vi "Actor Core.vi"(8 "error in":errorcluster, 11 "Batch proc":refnum<class "Batch Processor.lvclass">) -> (0 "error out":errorcluster, 3 "Actor out":refnum<class "Actor.lvclass">)   [LabVIEW 2016, in "Batch Processor.lvclass"]
doc: "LabActor main control pannel"
uses:
  Batch Processor.lvclass
  C:/Github/LabActor/Controllers/Application Controller/Application Controller.lvclass
  C:/Github/LabActor/Template Module/Template Module.lvclass
  C:/Program Files/National Instruments/LabVIEW 2016/vi.lib/ActorFramework/Actor/Actor.lvclass
  <vilib>/ActorFramework/Actor/Actor.lvclass
  NHMFL_Core/Libraries/Queued Listbox/Queued Listbox.xctl
  Application Controller/Application Controller.lvclass/Application Controller.ctl
  Template Module/Template Module.lvclass/Template Module.ctl
  <vilib>/ActorFramework/Actor/Actor.lvclass/Actor.ctl
  <vilib>/ActorFramework/Message Enqueuer/Message Enqueuer.lvclass/Message Enqueuer.ctl
  Batch Processor Messages/Start Batch Process Msg/Start Batch Process Msg.lvclass/Start Batch Process Msg.ctl
  <vilib>/Utility/sysdir.llb/System Directory Type.ctl
  Template Module Messages/Save Configuration Msg/Save Configuration Msg.lvclass/Save Configuration Msg.ctl
  Batch Processor Messages/List Folder Files Msg/List Folder Files Msg.lvclass/List Folder Files Msg.ctl
  Plots/Plot types.ctl
  Application Controller Messages/Open Waveform File Plot Msg/Open Waveform File Plot Msg.lvclass/Open Waveform File Plot Msg.ctl
  Monitor-Pulse Messages/Stop Measurements Command Msg/Stop Measurements Command Msg.lvclass/Stop Measurements Command Msg.ctl
  Application Controller/Write Monitor Running.vi
  Application Controller/Write Monitor ref.vi
  Application Controller/Write Start button.vi
  Application Controller/Write Stop button.vi
  Template Module/Read stop event.vi
  Application Controller/Read Monitor start event.vi
  Application Controller/Read Monitor stop event.vi
  Template Module/Read Open item event.vi
  Application Controller/Write Postproc ref.vi
  <vilib>/ActorFramework/Message Enqueuer/Init from Existing Queue.vi
  <vilib>/ActorFramework/Message Enqueuer/Enqueue.vi
  <vilib>/ActorFramework/Stop Msg/Stop Msg.lvclass
  C:/Program Files/National Instruments/LabVIEW 2016/vi.lib/ActorFramework/Message/Message.lvclass
  Batch Processor Messages/Start Batch Process Msg/Start Batch Process Msg.lvclass
  Template Module Messages/Save Configuration Msg/Save Configuration Msg.lvclass
  Batch Processor Messages/List Folder Files Msg/List Folder Files Msg.lvclass
  Application Controller Messages/Open Waveform File Plot Msg/Open Waveform File Plot Msg.lvclass
  Monitor-Pulse Messages/Stop Measurements Command Msg/Stop Measurements Command Msg.lvclass
  <vilib>/ActorFramework/Message Priority Queue/Priority Enqueue.vi
  Application Controller/Application Controller.lvclass
  <vilib>/ActorFramework/Message Enqueuer/Message Enqueuer.lvclass
  Template Module Messages/Restore Configuration Msg/Restore Configuration Msg.lvclass
panel:
  out "Elapsed time":dbl format="%#_gs"
  in  "Configuration":T1
  in  "All files in folder":bool
  in  "About Button":bool
  in  "Clear log":bool
  out "Error log":string
  out "Monitor file":path caption="Monitor\nFile"
  in  "Exit":bool
  in  "Write cfg":bool
  in  "Read cfg":bool
  in  "View XY Plot":bool
  out "Monitor Running":bool
  in  "Stop monitor":bool
  in  "Start monitor":bool
  in  "Monitor":string[](xcontrol) caption="Processors"
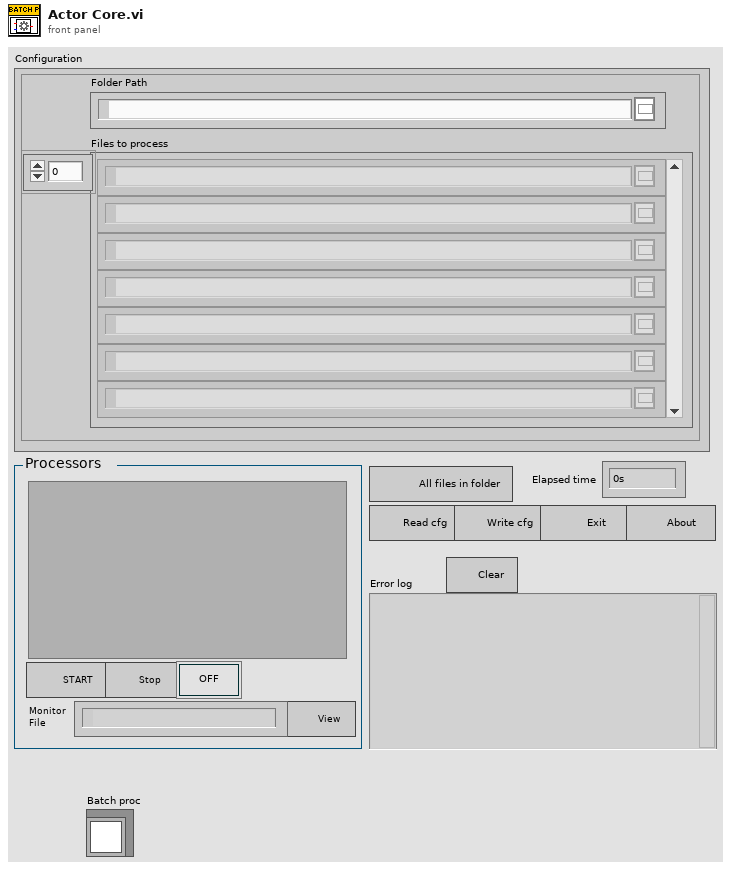
[diagram p1: front panel]
types:
  T1 = cluster{"Folder Path":path, "Files to process":path[]}
  T2 = typedef "Plot types.ctl" = enum16{"Waveform Plot", "XY Plot", "Full XY"}
  T3 = typedef "System Directory Type.ctl" = i32
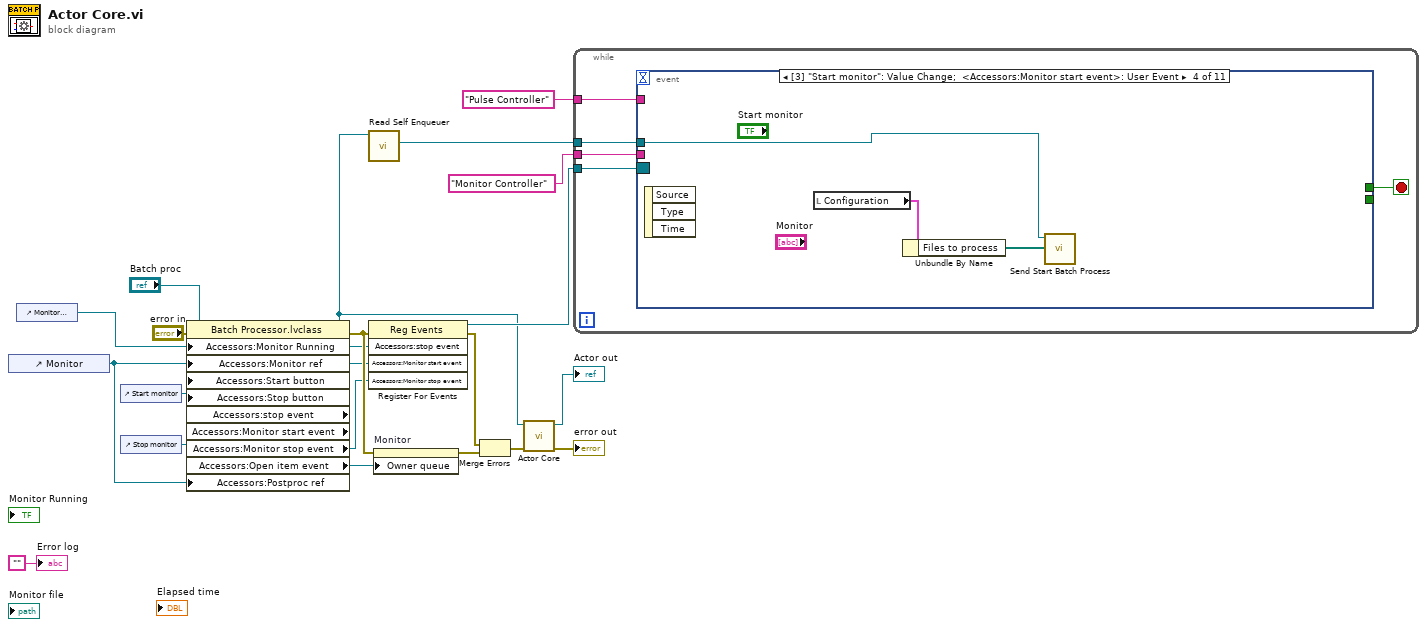
[diagram p0: block diagram]
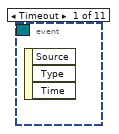
[diagram p2: hidden frame]
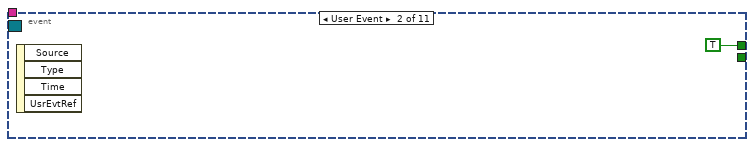
[diagram p3: hidden frame]
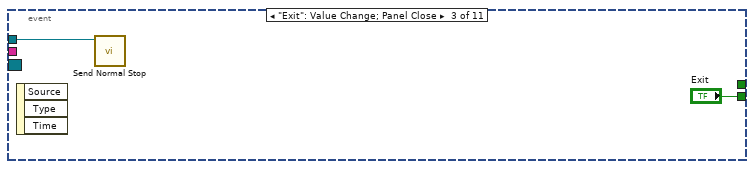
[diagram p4: hidden frame]
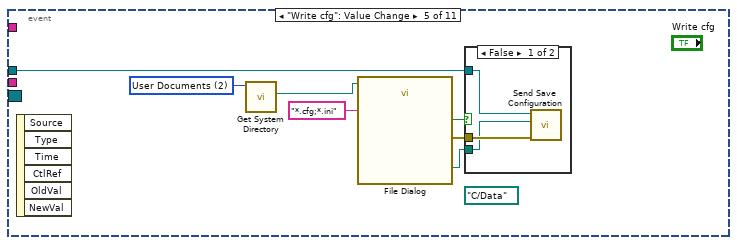
[diagram p5: hidden frame]
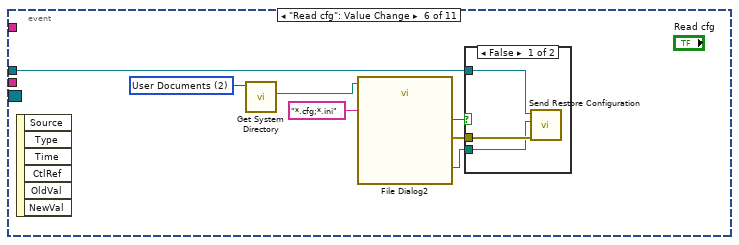
[diagram p7: hidden frame]
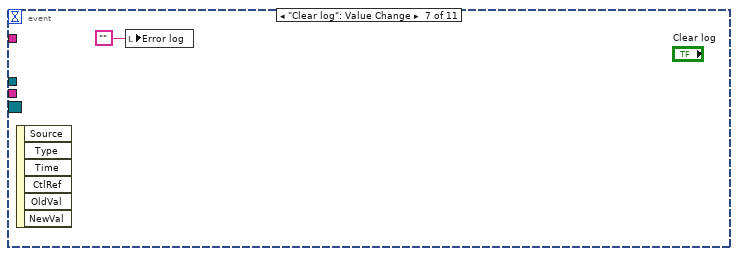
[diagram p9: hidden frame]
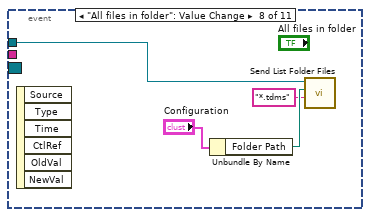
[diagram p10: hidden frame]
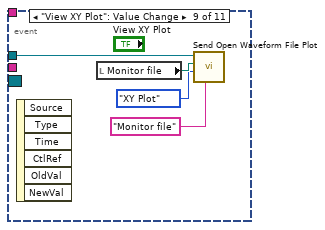
[diagram p11: hidden frame]
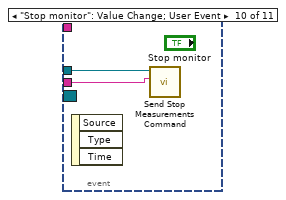
[diagram p12: hidden frame]
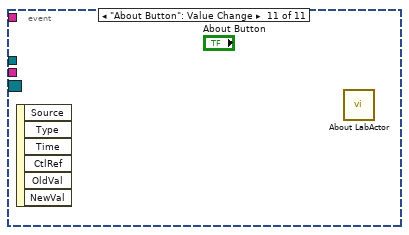
[diagram p13: hidden frame]
diagram:
  n1 = control-ref of="Monitor"() -> (w1:refnum<vi>)
  n2 = control-ref of="Monitor Running"() -> (w6:refnum<vi>)
  n3 = control-ref of="Start monitor"() -> (w4:refnum<vi>)
  n4 = control-ref of="Stop monitor"() -> (w5:refnum<vi>)
  n5 = property class="Batch Processor.lvclass"(reference="Batch proc", error in="error in", "Accessors:Monitor Running"=w6, "Accessors:Monitor ref"=w1, "Accessors:Start button"=w4, "Accessors:Stop button"=w5, "Accessors:Postproc ref"=w1) -> (reference out=w12:refnum<class "Batch Processor.lvclass">, error out=w16:errorcluster, "Accessors:stop event"=w7:refnum<user-event>, "Accessors:Monitor start event"=w3:refnum<user-event>, "Accessors:Monitor stop event"=w2:refnum<user-event>, "Accessors:Open item event"=w18:refnum<user-event>)
  n6 = call <vilib>:"Read Self Enqueuer.vi"("Actor"=w12) -> ("Self Enqueuer"=w11:refnum<class "Message Enqueuer.lvclass">)  [unwired: 10 in]
  n7 = register-events(error in=w16, w7, w3, w2) -> (reference out=w19:refnum<event-registration>, error out=w15:errorcluster)  [unwired: 1 in]
  n8 = property on="Monitor" class="Queued Listbox (strict)"(error in=w16, "Owner queue"=w18) -> (error out=w17:errorcluster)  [unwired: 1 in, 1 out]
  n9 = Merge Errors(w15, w17) -> (w13:errorcluster)
  n10 = call-parent "Actor Core.vi"("error in"=w13, "Measure Object in"=w12) -> ("error out"=→"error out":errorcluster, "Actor out"=→"Actor out":refnum<class "Actor.lvclass">)  [unwired: 8 in]
  n11 = while {
    tunnel: w19 -> [w27]
    tunnel: w11 -> [w25]
    tunnel: "Monitor Controller" ("Controller name") -> [w24]
    tunnel: "Pulse Controller" ("Item name") -> [w23]
    stop <- w26 stop-if-true
    n12 = event shown="[3] \"Start monitor\": Value Change;  <Accessors:Monitor start event>: User Event" {
      selector: w27 -> [_ _ _ _ _ _ _ _ _ _ _]
      dyn-events: _ -> [_ _ _ _ _ _ _ _ _ _ _]
      timeout: _ -> [_ _ _ _ _ _ _ _ _ _ _]
      tunnel: [_ TRUE _ _ _ _ _ _ _ _ _] -> w26
      tunnel: w25 -> [_ _ w29 w33 w37 w45 _ w58 w62 w64 _]
      tunnel: [_ _ "Exit" _ _ _ _ _ _ _ _] -> _
      tunnel: w24 -> [_ _ _ _ _ _ _ _ _ w63 _]
      tunnel: w23 -> [_ _ _ _ _ _ _ _ _ _ _]
      event Timeout {
        n13 = event-data() -> ()  [unwired: 1 in, 3 out]
      }
      event User Event {
        n14 = event-data() -> ()  [unwired: 1 in, 4 out]
      }
      event "Exit": Value Change; Panel Close {
        n15 = event-data() -> ()  [unwired: 1 in, 3 out]
        n16 = call <vilib>:"Send Normal Stop.vi"("Message Enqueuer"=w29) -> ()  [unwired: 10 in, 1 out]
      }
      event "Start monitor": Value Change; User Event {
        n17 = event-data() -> ()  [unwired: 1 in, 3 out]
        n18 = local read "Configuration"() -> (w32:T1)
        n19 = Unbundle By Name(w32) -> ("Files to process"=w31:path[])
        n20 = call "Send Start Batch Process.vi"("Files to process"=w31, "Message Enqueuer"=w33) -> ()  [unwired: 8 in, 2 out]
      }
      event "Write cfg": Value Change {
        w35 = T3 2 items=["User Home"=0, "User Desktop"=1, "User Documents"=2, "User Application Data"=3, "User Preferences"=4, "User Temporary"=5, "Public Documents"=6, "Public Application Data"=7, "Public Preferences"=8, "Public Cache"=13, "System Core Libraries"=9, "System Installed Libraries"=10, "Application Files"=11, "Boot Volume Root"=12] ("system directory type")
        (unwired) path "C:/Data" ("start path")
        n21 = event-data() -> ()  [unwired: 1 in, 6 out]
        n22 = call <vilib>:"Get System Directory.vi"("system directory type"=w35) -> ("system directory"=w34:path)  [unwired: 10 in]
        n23 = call "File Dialog"("start path"=w34, "pattern (all files)"="*.cfg;*.ini") -> ("selected path"=w39:path, "cancelled"=w40:bool, "error out"=w36:errorcluster)  [unwired: 10 in, 1 out]
        n24 = case shown="False" w40 {
          tunnel: w39 -> [w41 _]
          tunnel: w37 -> [w43 _]
          tunnel: w36 -> [w42 _]
          frame False {
            n25 = call "Send Save Configuration.vi"("error in (no error)"=w42, "File path"=w41, "Message Enqueuer"=w43) -> ()  [unwired: 7 in, 2 out]
          }
          frame True {
          }
        }
      }
      event "Read cfg": Value Change {
        w47 = T3 2 items=["User Home"=0, "User Desktop"=1, "User Documents"=2, "User Application Data"=3, "User Preferences"=4, "User Temporary"=5, "Public Documents"=6, "Public Application Data"=7, "Public Preferences"=8, "Public Cache"=13, "System Core Libraries"=9, "System Installed Libraries"=10, "Application Files"=11, "Boot Volume Root"=12] ("system directory type")
        n26 = event-data() -> ()  [unwired: 1 in, 6 out]
        n27 = call <vilib>:"Get System Directory.vi"("system directory type"=w47) -> ("system directory"=w46:path)  [unwired: 10 in]
        n28 = call "File Dialog2"("start path"=w46, "pattern (all files)"="*.cfg;*.ini") -> ("selected path"=w50:path, "cancelled"=w44:bool, "error out"=w48:errorcluster)  [unwired: 10 in, 1 out]
        n29 = case shown="False" w44 {
          tunnel: w50 -> [w51 _]
          tunnel: w45 -> [w53 _]
          tunnel: w48 -> [w52 _]
          frame False {
            n30 = call "Send Restore Configuration.vi"("error in (no error)"=w52, "File path"=w51, "Message Enqueuer"=w53) -> ()  [unwired: 7 in, 2 out]
          }
          frame True {
          }
        }
      }
      event "Clear log": Value Change {
        n31 = event-data() -> ()  [unwired: 1 in, 6 out]
        n32 = local write "Error log"("" ("Error log")) -> ()
      }
      event "All files in folder": Value Change {
        n33 = event-data() -> ()  [unwired: 1 in, 6 out]
        n34 = Unbundle By Name("Configuration") -> ("Folder Path"=w56:path)
        n35 = call "Send List Folder Files.vi"("Pattern"="*.tdms", "Folder Path"=w56, "Message Enqueuer"=w58) -> ()  [unwired: 7 in, 2 out]
      }
      event "View XY Plot": Value Change {
        n36 = event-data() -> ()  [unwired: 1 in, 6 out]
        n37 = local read "Monitor file"() -> (w61:path)
        n38 = call "Send Open Waveform File Plot.vi"("Plot group"="Monitor file" ("Control Name"), "Plot type"=Plot_types."XY Plot", "File Path Control"=w61, "Message Enqueuer"=w62) -> ()  [unwired: 6 in, 2 out]
      }
      event "Stop monitor": Value Change; User Event {
        n39 = event-data() -> ()  [unwired: 1 in, 3 out]
        n40 = call "Send Stop Measurements Command.vi"("Measurement Controller"=w63, "Message Enqueuer"=w64) -> ()  [unwired: 8 in, 2 out]
      }
      event "About Button": Value Change {
        n41 = event-data() -> ()  [unwired: 1 in, 6 out]
        n42 = call "About LabActor.vi"() -> ()  [unwired: 12 in]
      }
    }
  }
  "Error log" <- "" ("Error log")
